vi "route_old_1.vi"(8 "error in (no error)":errorcluster, 9 "now position":cluster{"x":dbl, "y":dbl, "degree":dbl}, 11 "Enum":T1) -> (0 "error out":errorcluster, 1 "position out":cluster{"x":dbl, "y":dbl, "degree":dbl})   [LabVIEW 2019]
uses:
  20220212-contest/ctl/move.ctl
  ctl/continued move array-V2.ctl
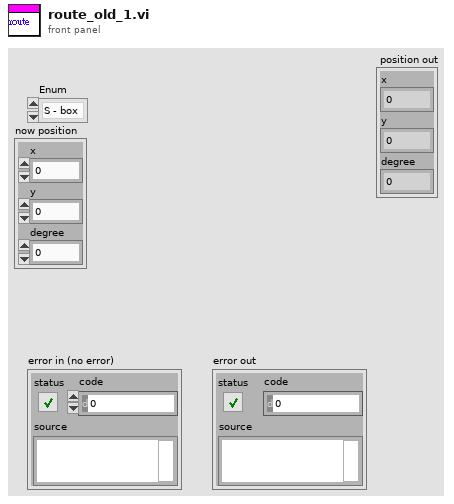
[diagram p1: front panel]
types:
  T1 = typedef "move.ctl" = enum16{"S - box", "box - R1", "R1 - box", "box - R2", "R2 - box", "box - R3", "R3 - box", "box - R4", "R4 - box", "box - R5", "R5 - box", "box - rec", "rec - box", "box - S", "box align", "box end"}
  T2 = typedef "continued move array-V2.ctl" = cluster{"X":dbl, "Y":dbl, "Speed":dbl, "rotate\ndegree":dbl, "deg":dbl}
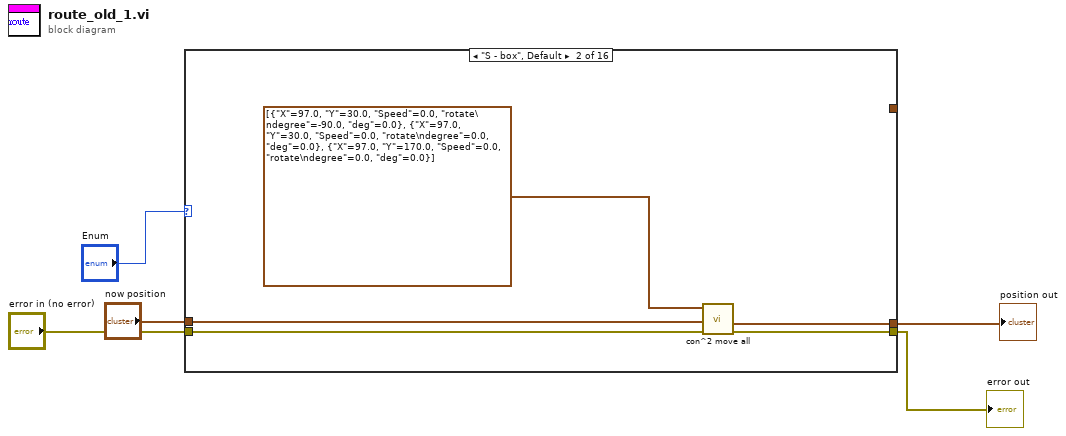
[diagram p0: block diagram]
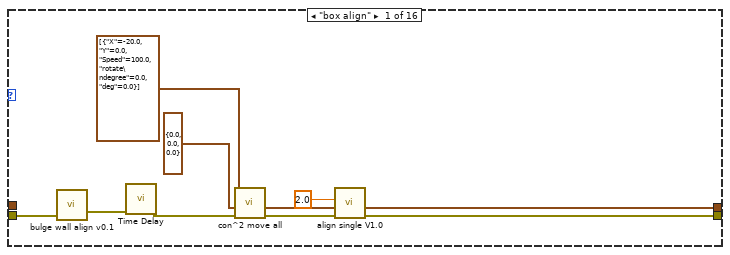
[diagram p2: hidden frame]
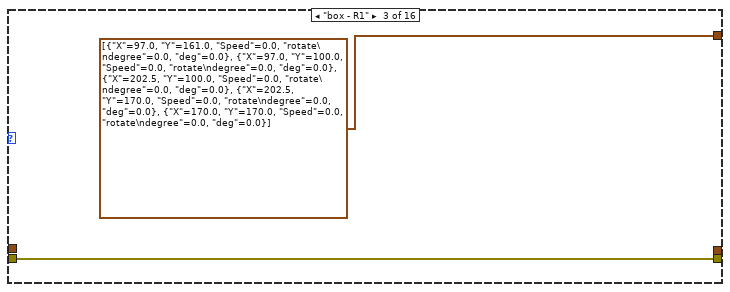
[diagram p3: hidden frame]
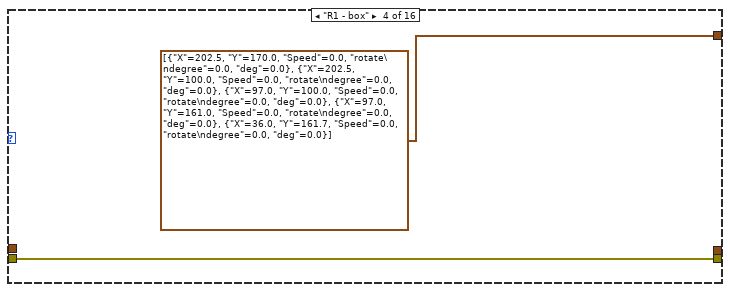
[diagram p4: hidden frame]
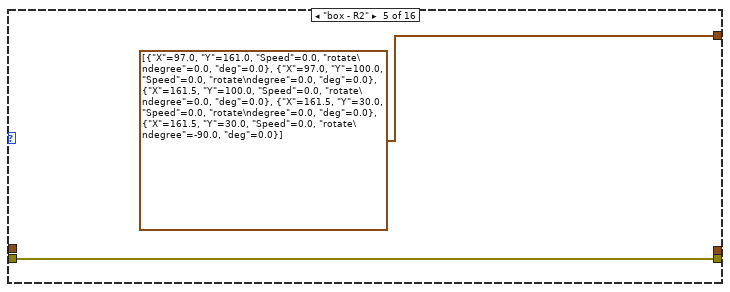
[diagram p5: hidden frame]
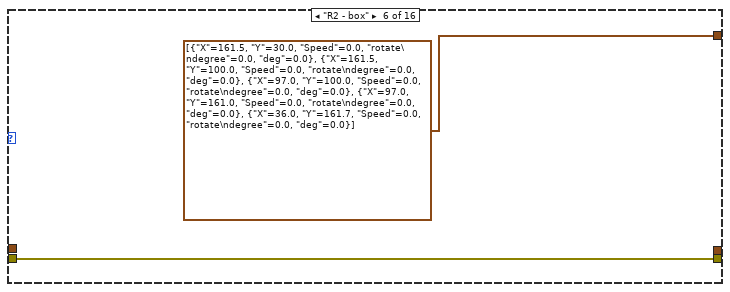
[diagram p6: hidden frame]
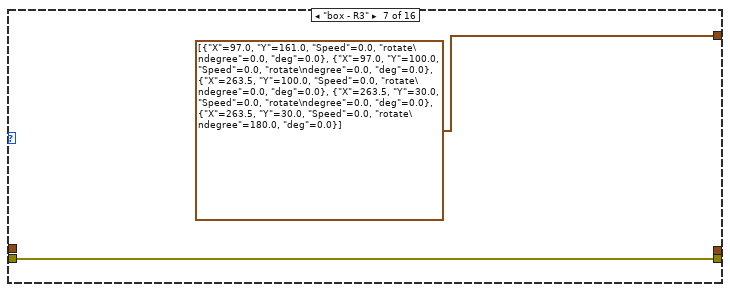
[diagram p7: hidden frame]
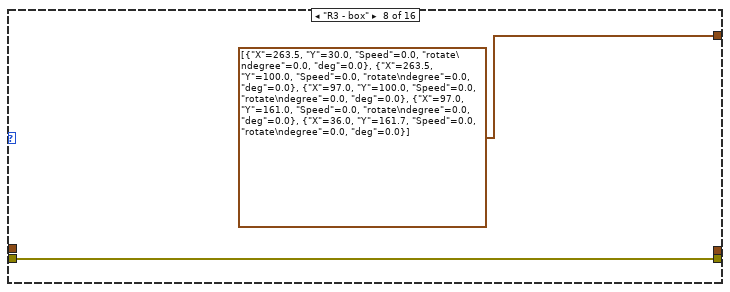
[diagram p8: hidden frame]
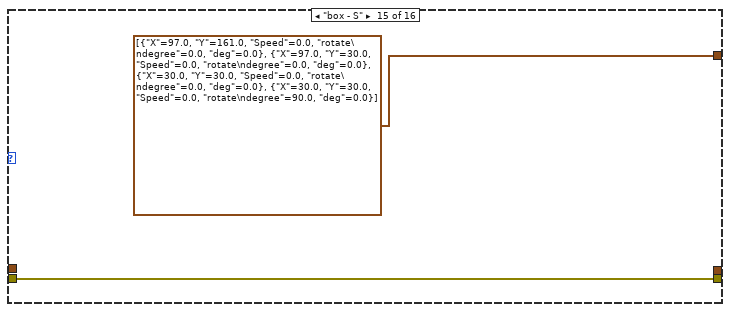
[diagram p15: hidden frame]
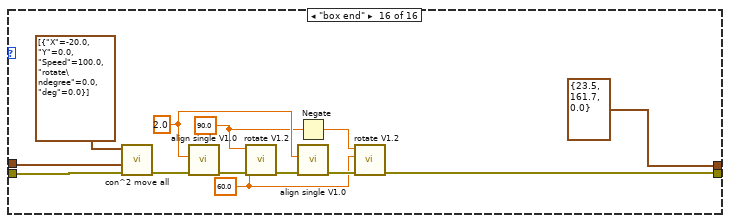
[diagram p16: hidden frame]
diagram:
  n1 = case shown="\"S - box\", Default" "Enum" {
    tunnel: [_ _ T2[] [{"X"=97.0, "Y"=161.0, "Speed"=0.0, "rotate\ndegree"=0.0, "deg"=0.0}, {"X"=97.0, "Y"=100.0, "Speed"=0.0, "rotate\ndegree"=0.0, "deg"=0.0}, {"X"=202.5, "Y"=100.0, "Speed"=0.0, "rotate\ndegree"=0.0, "deg"=0.0}, {"X"=202.5, "Y"=170.0, "Speed"=0.0, "rotate\ndegree"=0.0, "deg"=0.0}, {"X"=170.0, "Y"=170.0, "Speed"=0.0, "rotate\ndegree"=0.0, "deg"=0.0}] ("contrast move array") T2[] [{"X"=202.5, "Y"=170.0, "Speed"=0.0, "rotate\ndegree"=0.0, "deg"=0.0}, {"X"=202.5, "Y"=100.0, "Speed"=0.0, "rotate\ndegree"=0.0, "deg"=0.0}, {"X"=97.0, "Y"=100.0, "Speed"=0.0, "rotate\ndegree"=0.0, "deg"=0.0}, {"X"=97.0, "Y"=161.0, "Speed"=0.0, "rotate\ndegree"=0.0, "deg"=0.0}, {"X"=36.0, "Y"=161.7, "Speed"=0.0, "rotate\ndegree"=0.0, "deg"=0.0}] ("contrast move array") T2[] [{"X"=97.0, "Y"=161.0, "Speed"=0.0, "rotate\ndegree"=0.0, "deg"=0.0}, {"X"=97.0, "Y"=100.0, "Speed"=0.0, "rotate\ndegree"=0.0, "deg"=0.0}, {"X"=161.5, "Y"=100.0, "Speed"=0.0, "rotate\ndegree"=0.0, "deg"=0.0}, {"X"=161.5, "Y"=30.0, "Speed"=0.0, "rotate\ndegree"=0.0, "deg"=0.0}, {"X"=161.5, "Y"=30.0, "Speed"=0.0, "rotate\ndegree"=-90.0, "deg"=0.0}] ("contrast move array") T2[] [{"X"=161.5, "Y"=30.0, "Speed"=0.0, "rotate\ndegree"=0.0, "deg"=0.0}, {"X"=161.5, "Y"=100.0, "Speed"=0.0, "rotate\ndegree"=0.0, "deg"=0.0}, {"X"=97.0, "Y"=100.0, "Speed"=0.0, "rotate\ndegree"=0.0, "deg"=0.0}, {"X"=97.0, "Y"=161.0, "Speed"=0.0, "rotate\ndegree"=0.0, "deg"=0.0}, {"X"=36.0, "Y"=161.7, "Speed"=0.0, "rotate\ndegree"=0.0, "deg"=0.0}] ("contrast move array") T2[] [{"X"=97.0, "Y"=161.0, "Speed"=0.0, "rotate\ndegree"=0.0, "deg"=0.0}, {"X"=97.0, "Y"=100.0, "Speed"=0.0, "rotate\ndegree"=0.0, "deg"=0.0}, {"X"=263.5, "Y"=100.0, "Speed"=0.0, "rotate\ndegree"=0.0, "deg"=0.0}, {"X"=263.5, "Y"=30.0, "Speed"=0.0, "rotate\ndegree"=0.0, "deg"=0.0}, {"X"=263.5, "Y"=30.0, "Speed"=0.0, "rotate\ndegree"=180.0, "deg"=0.0}] ("contrast move array") T2[] [{"X"=263.5, "Y"=30.0, "Speed"=0.0, "rotate\ndegree"=0.0, "deg"=0.0}, {"X"=263.5, "Y"=100.0, "Speed"=0.0, "rotate\ndegree"=0.0, "deg"=0.0}, {"X"=97.0, "Y"=100.0, "Speed"=0.0, "rotate\ndegree"=0.0, "deg"=0.0}, {"X"=97.0, "Y"=161.0, "Speed"=0.0, "rotate\ndegree"=0.0, "deg"=0.0}, {"X"=36.0, "Y"=161.7, "Speed"=0.0, "rotate\ndegree"=0.0, "deg"=0.0}] ("contrast move array") _ _ _ _ _ _ T2[] [{"X"=97.0, "Y"=161.0, "Speed"=0.0, "rotate\ndegree"=0.0, "deg"=0.0}, {"X"=97.0, "Y"=30.0, "Speed"=0.0, "rotate\ndegree"=0.0, "deg"=0.0}, {"X"=30.0, "Y"=30.0, "Speed"=0.0, "rotate\ndegree"=0.0, "deg"=0.0}, {"X"=30.0, "Y"=30.0, "Speed"=0.0, "rotate\ndegree"=90.0, "deg"=0.0}] ("contrast move array") _] -> _
    tunnel: "error in (no error)" -> [w13 w18 w20 w22 w24 w26 w28 w30 w32 w33 w34 w35 w36 w37 w38 w52]
    tunnel: [w7 w19 w20 w22 w24 w26 w28 w30 w32 w33 w34 w35 w36 w37 w38 w41] -> w5
    tunnel: "now position" -> [_ w16 _ _ _ _ _ _ _ _ _ _ _ _ _ w51]
    tunnel: [w10 w15 _ _ _ _ _ _ _ _ _ _ _ _ _ cluster{"x":dbl, "y":dbl, "degree":dbl} {"x"=23.5, "y"=161.7, "degree"=0.0} ("position out")] -> w1
    frame "box align" {
      n2 = call "bulge wall align v0.1.vi"("error in (no error)"=w13) -> ("error out"=w9:errorcluster)  [unwired: 9 in, 1 out]
      n3 = call "Time Delay"("error in (no error)"=w9) -> ("error out"=w6:errorcluster)  [unwired: 10 in]
      n4 = call "con^2 move all.vi"("error in (no error)"=w6, "now position"=cluster{"x":dbl, "y":dbl, "degree":dbl} {"x"=0.0, "y"=0.0, "degree"=0.0} ("position out"), "contrast move array"=T2[] [{"X"=-20.0, "Y"=0.0, "Speed"=100.0, "rotate\ndegree"=0.0, "deg"=0.0}]) -> ("error out"=w8:errorcluster, "position out"=w10:cluster{"x":dbl, "y":dbl, "degree":dbl})  [unwired: 7 in]
      n5 = call "align single V1.0.vi"("error in (no error)"=w8, "Target (Volt)"=2.0) -> ("error out"=w7:errorcluster)  [unwired: 9 in]
    }
    frame "S - box", Default {
      n6 = call "con^2 move all.vi"("error in (no error)"=w18, "now position"=w16, "contrast move array"=T2[] [{"X"=97.0, "Y"=30.0, "Speed"=0.0, "rotate\ndegree"=-90.0, "deg"=0.0}, {"X"=97.0, "Y"=30.0, "Speed"=0.0, "rotate\ndegree"=0.0, "deg"=0.0}, {"X"=97.0, "Y"=170.0, "Speed"=0.0, "rotate\ndegree"=0.0, "deg"=0.0}]) -> ("error out"=w19:errorcluster, "position out"=w15:cluster{"x":dbl, "y":dbl, "degree":dbl})  [unwired: 7 in]
    }
    frame "box - R1" {
    }
    frame "R1 - box" {
    }
    frame "box - R2" {
    }
    frame "R2 - box" {
    }
    frame "box - R3" {
    }
    frame "R3 - box" {
    }
    frame "box - R4" {
    }
    frame "R4 - box" {
    }
    frame "box - R5" {
    }
    frame "R5 - box" {
    }
    frame "box - rec" {
    }
    frame "rec - box" {
    }
    frame "box - S" {
    }
    frame "box end" {
      w44 = 60.0 ("speed")
      w42 = 90.0 ("degree")
      w46 = 2.0 ("Target (Volt)")
      n7 = call "con^2 move all.vi"("error in (no error)"=w52, "now position"=w51, "contrast move array"=T2[] [{"X"=-20.0, "Y"=0.0, "Speed"=100.0, "rotate\ndegree"=0.0, "deg"=0.0}]) -> ("error out"=w49:errorcluster)  [unwired: 7 in, 1 out]
      n8 = call "align single V1.0.vi"("error in (no error)"=w49, "Target (Volt)"=w46) -> ("error out"=w48:errorcluster)  [unwired: 9 in]
      n9 = call "rotate V1.2.vi"("error in (no error)"=w48, "speed"=w44, "degree"=w42) -> ("error out"=w47:errorcluster)  [unwired: 8 in]
      n10 = Negate(x=w42) -> (-x=w43:dbl)
      n11 = call "align single V1.0.vi"("error in (no error)"=w47, "Target (Volt)"=w46) -> ("error out"=w45:errorcluster)  [unwired: 9 in]
      n12 = call "rotate V1.2.vi"("error in (no error)"=w45, "speed"=w44, "degree"=w43) -> ("error out"=w41:errorcluster)  [unwired: 8 in]
    }
  }
  "error out" <- w5
  "position out" <- w1
